vi "Desktop Main.vi"() -> ()   [LabVIEW 2021]
doc: "Demonstrates the use of Transmission Control Protocol (TCP) to communicate between the host computer and one or multiple myRIO targets."
uses:
  Sub VIs/State Info.ctl
  Sub VIs/Connection Info.ctl
panel:
  in  "LED":bool[](array[boolean])=[FALSE, FALSE, FALSE, FALSE]
  out "error out":errorcluster
  out "Number of Client Connections":i32
  in  "Stop":bool
  # "Overview: Demonstrates the use of Transmission Control Protocol (TCP) to communicate between the host computer and one or multiple myRIO targets.\nInstructions:\n1. Run this VI.\n2. Open RT Main.vi and follow its front panel instructions.\n3. Change the value of LED and observe the LEDs on the myRIO device and the value of LED Status on RT Main.vi. They change when the value of LED on this VI changes.\n4. Click Stop to stop this VI."
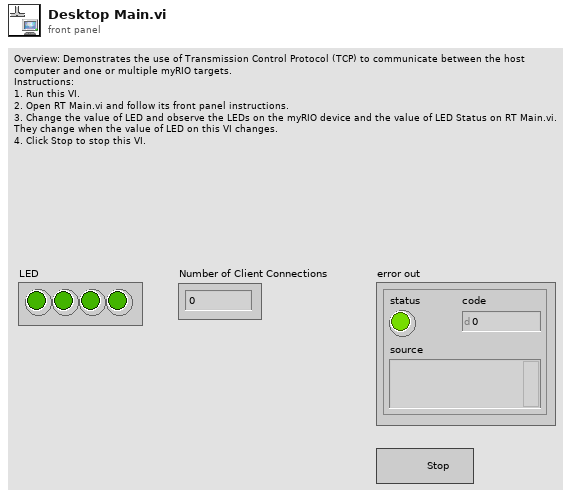
[diagram p1: front panel]
types:
  T1 = typedef "Connection Info.ctl" = cluster{"All Clients":cluster{"TCP Connection Refnum":refnum<k5>, "Connection Name":string}[], "Listener":refnum<k5>}
  T2 = typedef "State Info.ctl" = enum16{"Initialize", "Status Check", "Process", "Stop"}
  T3 = cluster{"TCP Connection Refnum":refnum<k5>, "Name":string}
  T4 = cluster{"TCP Connection Refnum":refnum<k5>, "Connection Name":string}[]
  T5 = cluster{"TCP Connection Refnum":refnum<k5>, "Name":string}[]
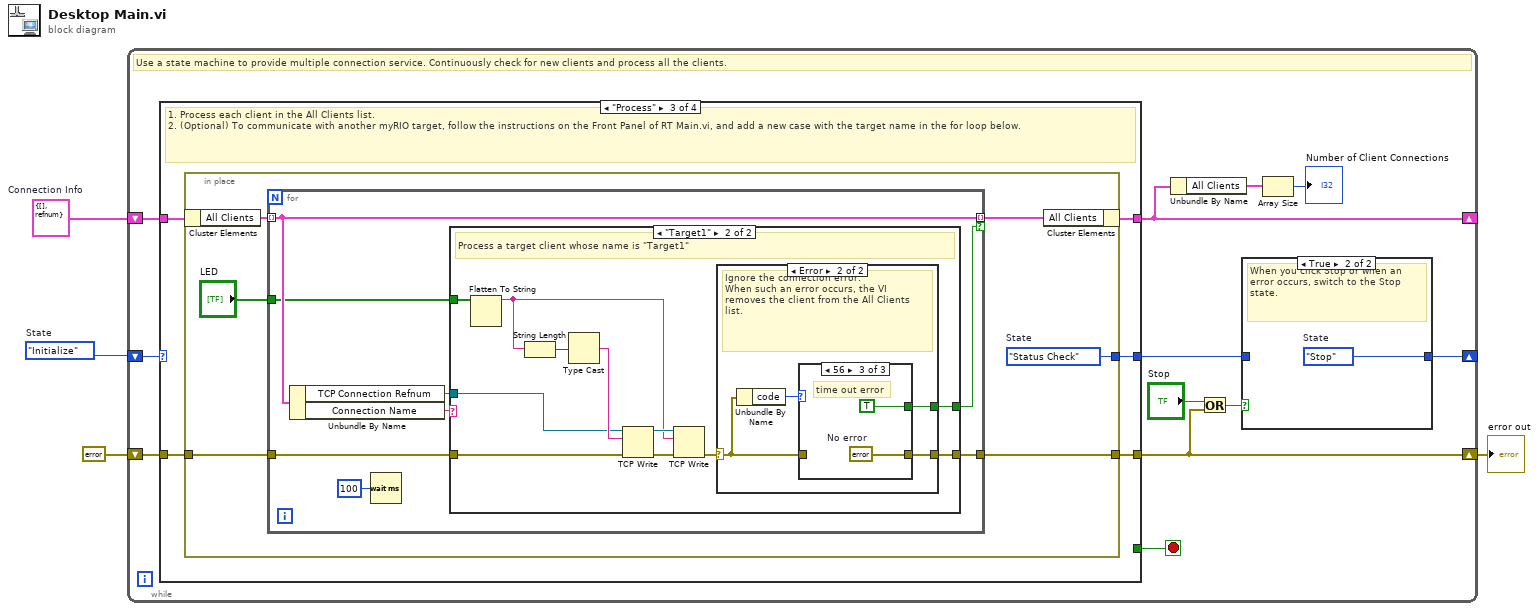
[diagram p0: block diagram]
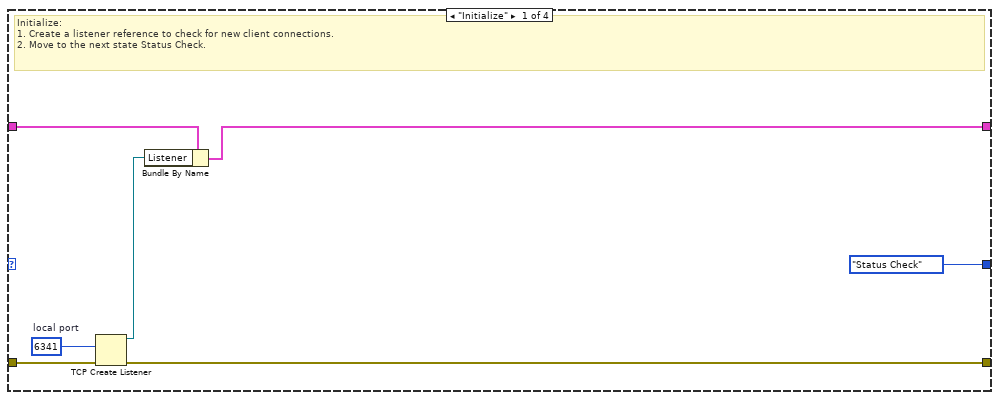
[diagram p3: hidden frame]
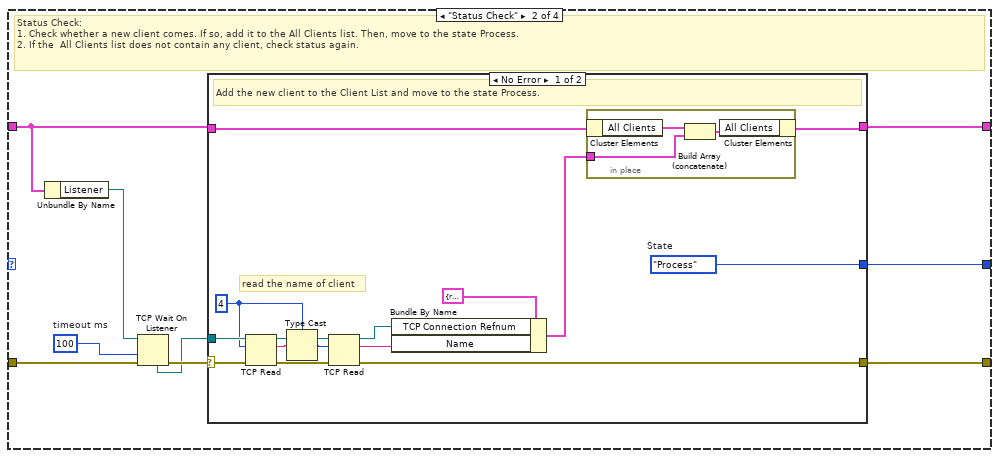
[diagram p4: hidden frame]
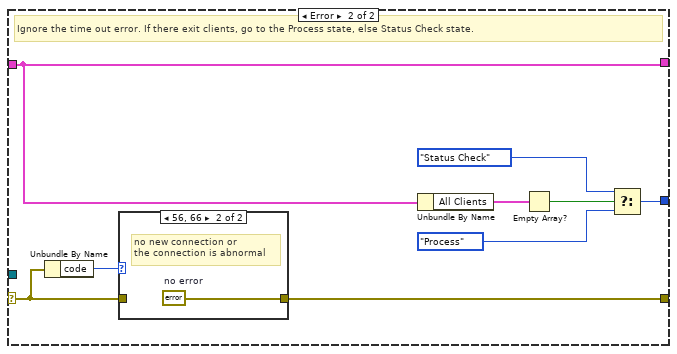
[diagram p5: hidden frame]
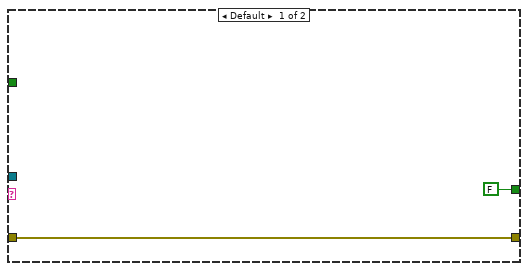
[diagram p7: hidden frame]
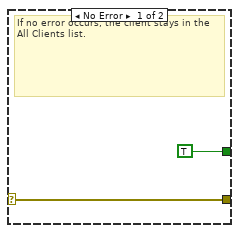
[diagram p8: hidden frame]
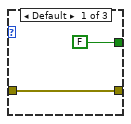
[diagram p9: hidden frame]
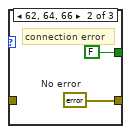
[diagram p10: hidden frame]
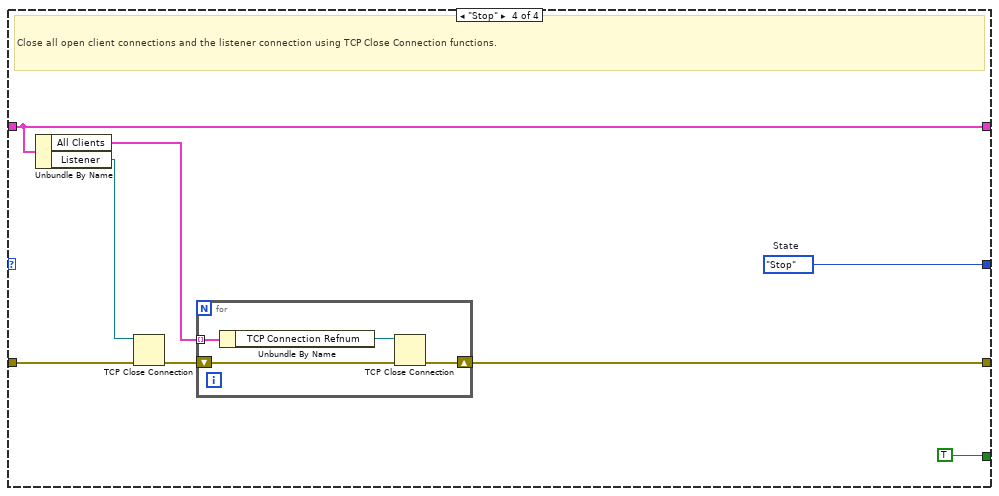
[diagram p11: hidden frame]
diagram:
  w3 = T1 {"All Clients"=[], "Listener"=refnum}  # Connection Info
  w2 = State_Info."Initialize"  # State
  n1 = while {
    shift-right: [w8] -> _
    shift-left: w3 -> [w16]
    shift-right: [w5] -> w1
    shift-left: errorcluster {"status"=FALSE, "code"=0, "source"=""} ("error in (no error)") -> [w15]
    shift-right: [w12] -> _
    shift-left: w2 -> [w9]
    stop <- w14 stop-if-true
    # "Use a state machine to provide multiple connection service. Continuously check for new clients and process all the clients."
    n2 = case shown="\"Process\"" w9 {
      tunnel: w16 -> [w24 w31 w68 w110]
      tunnel: w15 -> [w25 w32 w67 w112]
      tunnel: [w22 w28 w65 w110] -> w8
      tunnel: [w21 w29 w64 w108] -> w5
      tunnel: [State_Info."Status Check" w30 w66 w109] -> w13
      tunnel: [_ _ _ TRUE] -> w14
      frame "Initialize" {
        w19 = u16 6341  # local port
        # "Initialize:\n1. Create a listener reference to check for new client connections.\n2. Move to the next state Status Check."
        n3 = TCP Create Listener(8:w25, 10:w19) -> (0:w21:errorcluster, 3:w23:refnum<k5>)  [unwired: 4 out]
        n4 = Bundle By Name(cluster=w24, "Listener"=w23) -> (w22:T1)
      }
      frame "Status Check" {
        w34 = 100  # timeout ms
        # "Status Check:\n1. Check whether a new client comes. If so, add it to the All Clients list. Then, move to the state Process.\n2. If the  All Clients list does not contain any client, check status again."
        n5 = Unbundle By Name(w31) -> ("Listener"=w33:refnum<k5>)
        n6 = TCP Wait On Listener(8:w32, 9:w34, 11:w33) -> (0:w27:errorcluster, 4:w26:refnum<k5>)  [unwired: 4 out]
        n7 = case shown="No Error" w27 {
          selector: w27 -> [w42 w60]
          tunnel: w31 -> [w47 w57]
          tunnel: [w49 w55] -> w30
          tunnel: [w48 w57] -> w28
          tunnel: [w36 w56] -> w29
          tunnel: w26 -> [w41 _]
          frame No Error {
            w38 = 4 ("bytes to read")
            w49 = State_Info."Process"  # State
            # "read the name of client"
            # "Add the new client to the Client List and move to the state Process."
            n8 = TCP Read(connection ID=w41, bytes to read=w38, error in (no error)=w42) -> (connection ID out=w43:refnum<k5>, data out=w39:string, error out=w44:errorcluster)  [unwired: 2 in]
            n9 = Type Cast(type=w38, x=w39) -> (*(type *) &x=w37:i32)
            n10 = TCP Read(connection ID=w43, bytes to read=w37, error in (no error)=w44) -> (connection ID out=w40:refnum<k5>, data out=w35:string, error out=w36:errorcluster)  [unwired: 2 in]
            n11 = Bundle By Name(cluster=T3 {"TCP Connection Refnum"=refnum, "Name"=""} ("Client"), "TCP Connection Refnum"=w40, "Name"=w35) -> (w46:T3)
            n12 = in-place {
              in-place-border: w46 -> [w51]
              n13 = in-place-cluster #1(w47) -> ("All Clients"=w52:T4)
              n14 = Build Array (concatenate)(w52, w51) -> (w50:T5)
              n15 = in-place-cluster #1("All Clients"=w50) -> (w48:T1)
            }
          }
          frame Error {
            # "Ignore the time out error. If there exit clients, go to the Process state, else Status Check state."
            n16 = Unbundle By Name(w60) -> ("code"=w61:i32)
            n17 = case shown="56, 66" w61 {
              tunnel: w60 -> [w62 _]
              tunnel: [w62 w63] -> w56
              frame Default {
              }
              frame 56, 66 {
                w63 = errorcluster {"status"=FALSE, "code"=0, "source"=""}  # no error
                # "no new connection or\nthe connection is abnormal"
              }
            }
            n18 = Unbundle By Name(w57) -> ("All Clients"=w59:T4)
            n19 = Empty Array?(array=w59) -> (empty?=w58:bool)
            n20 = Select(t=State_Info."Status Check" ("Initial State"), s=w58, f=State_Info."Process" ("Initial State")) -> (s? t:f=w55:T2)
          }
        }
      }
      frame "Process" {
        # "1. Process each client in the All Clients list.\n2. (Optional) To communicate with another myRIO target, follow the instructions on the Front Panel of RT Main.vi, and add a new case with the target name in the for loop below."
        n21 = in-place {
          in-place-border: w67 -> [w71]
          in-place-border: [w74] -> w66
          in-place-border: [w70] -> w64
          w74 = State_Info."Status Check"  # State
          n22 = in-place-cluster #2(w68) -> ("All Clients"=w73:T4)
          n23 = for {
            tunnel: w73 -> [w80] mode=indexing
            tunnel: [w80] -> w72 mode=indexing if=w76
            tunnel: "LED" -> [w78]
            tunnel: w71 -> [w77]
            tunnel: [w75] -> w70
            n24 = Unbundle By Name(w80) -> ("TCP Connection Refnum"=w81:refnum<k5>, "Connection Name"=w82:string)
            n25 = Wait (ms)(milliseconds to wait=u32 100) -> ()  [unwired: 1 out]
            n26 = case shown="\"Target1\"" w82 {
              tunnel: w81 -> [_ w92]
              tunnel: w78 -> [_ w93]
              tunnel: w77 -> [w83 w91]
              tunnel: [FALSE w87] -> w76
              tunnel: [w83 w85] -> w75
              frame Default {
              }
              frame "Target1" {
                # "Process a target client whose name is \"Target1\""
                n27 = Flatten To String(anything=w93) -> (data string=w88:string)  [unwired: 3 in, 2 out]
                n28 = String Length(string=w88) -> (length=w95:i32)
                n29 = Type Cast(x=w95) -> (*(type *) &x=w94:string)  [unwired: 1 in]
                n30 = TCP Write(connection ID=w92, data in=w94, error in (no error)=w91) -> (connection ID out=w89:refnum<k5>, error out=w90:errorcluster)  [unwired: 1 in, 1 out]
                n31 = TCP Write(connection ID=w89, data in=w88, error in (no error)=w90) -> (error out=w86:errorcluster)  [unwired: 1 in, 2 out]
                n32 = case shown="Error" w86 {
                  selector: w86 -> [w97 w100]
                  tunnel: [TRUE w98] -> w87
                  tunnel: [w97 w99] -> w85
                  frame No Error {
                    # "If no error occurs, the client stays in the All Clients list."
                  }
                  frame Error {
                    # "Ignore the connection error.\nWhen such an error occurs, the VI removes the client from the All Clients list."
                    n33 = Unbundle By Name(w100) -> ("code"=w101:i32)
                    n34 = case shown="56" w101 {
                      tunnel: w100 -> [w103 _ _]
                      tunnel: [w103 w104 w106] -> w99
                      tunnel: [FALSE FALSE TRUE] -> w98
                      frame Default {
                      }
                      frame 62, 64, 66 {
                        w104 = errorcluster {"status"=FALSE, "code"=0, "source"=""}  # No error
                        # "connection error"
                      }
                      frame 56 {
                        w106 = errorcluster {"status"=FALSE, "code"=0, "source"=""}  # No error
                        # "time out error"
                      }
                    }
                  }
                }
              }
            }
          }
          n35 = in-place-cluster #2("All Clients"=w72) -> (w65:T1)
        }
      }
      frame "Stop" {
        w109 = State_Info."Stop"  # State
        # "Close all open client connections and the listener connection using TCP Close Connection functions."
        n36 = Unbundle By Name(w110) -> ("All Clients"=w113:T4, "Listener"=w114:refnum<k5>)
        n37 = TCP Close Connection(connection ID=w114, error in (no error)=w112) -> (error out=w115:errorcluster)  [unwired: 1 in, 1 out]
        n38 = for {
          shift-right: [w118] -> w108
          shift-left: w115 -> [w119]
          tunnel: w113 -> [w117] mode=indexing
          n39 = Unbundle By Name(w117) -> ("TCP Connection Refnum"=w116:refnum<k5>)
          n40 = TCP Close Connection(connection ID=w116, error in (no error)=w119) -> (error out=w118:errorcluster)  [unwired: 1 in, 1 out]
        }
      }
    }
    n41 = Unbundle By Name(w8) -> ("All Clients"=w6:T4)
    n42 = Or(x="Stop", y=w5) -> (x .or. y?=w10:bool)
    n43 = case shown="True" w10 {
      tunnel: w13 -> [w17 _]
      tunnel: [w17 w18] -> w12
      frame False {
      }
      frame True {
        w18 = State_Info."Stop"  # State
        # "When you click Stop or when an error occurs, switch to the Stop state."
      }
    }
    n44 = Array Size(array=w6) -> (size(s)=→"Number of Client Connections":i32)
  }
  "error out" <- w1
